vi "Main.vi"() -> ()   [LabVIEW 2010]
uses:
  <vilib>/Utility/inputDevices.llb/closeKeyboard.vi
  <vilib>/Utility/inputDevices.llb/keyboardAcquire.vi
panel:
  in  "Tab":enum32{"Load"}(tab)
  out "loading":u16(ring)
  in  "game show tab":T1(tab)=enum."Method"
  in  "Game Start":bool
  in  "Game Caption":bool
  in  "Game Restart":bool
  in  "String":string="1.按“SPACE”跳跃；\n2.按“SHIFT+SPACE”穿越障碍物！"
  in  "Game Sound":bool=TRUE
  in  "Game Pause":bool
  out "Load-I":i32=60
  in  "Game Close":bool
  in  "Game Slide":dbl(slide) scale=0.0..6.0
  in  "error in (no error)":errorcluster
  in  "MAP2":T2={"Game Road 1"=1, "Game Road 2"=1, "Game Road 3"=0, "Game Road 4"=1, "Game Road 5"=1, "Game Road 6"=1, "Game Road 7"=2, "Game Road 8"=1, "Game Road 9"=1, "Game Road 10"=1, "Game Road 11"=1, "Game Road 12"=1, "Game Road 13"=1, "Game Road 14"=1, "Game Road 15"=0, "Game Coin 1"=1, "Game Coin 2"=1, "Game Coin 3"=1, "Game Coin 4"=1, "Game Coin 5"=1, "Game Coin 6"=1, "Game Coin 7"=1, "Game Coin 8"=1, "Game Coin 9"=2, "Game Coin 10"=2, "Game Coin 11"=2, "Game Coin 12"=2, "Game Coin 13"=1, "Game Coin 14"=1, "Game Coin 15"=1, "Game Coin 16"=1, "Game Coin 17"=1, "Game Coin 18"=1, "Game Coin 19"=1, "Game Coin 20"=1, "Game Coin 21"=2, "Game Coin 22"=2, "Game Coin 23"=2, "Game Coin 24"=2, "Game Coin 25"=2, "Game Coin 26"=2, "Game Coin 27"=2, "Game Coin 28"=2, "Game Coin 29"=2, "Game Coin 30"=2, "Game Coin 31"=2, "Game Coin 32"=2, "Game Coin 33"=1, "Game Coin 34"=1, "Game Coin 35"=1, "Game Coin 36"=1, "Game Coin 37"=1, "Game Coin 38"=1, "Game Coin 39"=1, "Game Coin 40"=1, "Game Coin 41"=1, "Game Coin 42"=1, "Game Coin 43"=1, "Game Coin 44"=1, "Game Coin 45"=1, "Game Coin 46"=1, "Game Coin 47"=1, "Game Coin 48"=1, "Game Coin 49"=1, "Game Coin 50"=1, "Game Coin 51"=2, "Game Coin 52"=2, "Game Coin 53"=2, "Game Coin 54"=2, "Game Coin 55"=2, "Game Coin 56"=2, "Game Coin 57"=2, "Game Coin 58"=2, "Game Coin 59"=2, "Game Coin 60"=2}
  in  "Game Cat":u16(ring)=1
  out "Bool":bool
  in  "music":refnum<k7>(container)
  in  "background_music":refnum<k7>(container)
  in  "Score":u16[](array[ring])=[0, 0, 0, 0, 0, 0, 0, 0]
  in  "MAP1":T2={"Game Road 1"=1, "Game Road 2"=1, "Game Road 3"=1, "Game Road 4"=1, "Game Road 5"=1, "Game Road 6"=1, "Game Road 7"=0, "Game Road 8"=1, "Game Road 9"=1, "Game Road 10"=1, "Game Road 11"=1, "Game Road 12"=2, "Game Road 13"=1, "Game Road 14"=1, "Game Road 15"=0, "Game Coin 1"=0, "Game Coin 2"=0, "Game Coin 3"=0, "Game Coin 4"=0, "Game Coin 5"=1, "Game Coin 6"=1, "Game Coin 7"=1, "Game Coin 8"=1, "Game Coin 9"=1, "Game Coin 10"=1, "Game Coin 11"=1, "Game Coin 12"=1, "Game Coin 13"=1, "Game Coin 14"=1, "Game Coin 15"=1, "Game Coin 16"=1, "Game Coin 17"=1, "Game Coin 18"=1, "Game Coin 19"=1, "Game Coin 20"=1, "Game Coin 21"=1, "Game Coin 22"=1, "Game Coin 23"=1, "Game Coin 24"=2, "Game Coin 25"=2, "Game Coin 26"=2, "Game Coin 27"=2, "Game Coin 28"=2, "Game Coin 29"=2, "Game Coin 30"=1, "Game Coin 31"=1, "Game Coin 32"=1, "Game Coin 33"=1, "Game Coin 34"=1, "Game Coin 35"=1, "Game Coin 36"=1, "Game Coin 37"=1, "Game Coin 38"=1, "Game Coin 39"=1, "Game Coin 40"=2, "Game Coin 41"=2, "Game Coin 42"=2, "Game Coin 43"=2, "Game Coin 44"=1, "Game Coin 45"=1, "Game Coin 46"=1, "Game Coin 47"=1, "Game Coin 48"=1, "Game Coin 49"=1, "Game Coin 50"=2, "Game Coin 51"=2, "Game Coin 52"=2, "Game Coin 53"=2, "Game Coin 54"=2, "Game Coin 55"=2, "Game Coin 56"=2, "Game Coin 57"=2, "Game Coin 58"=2, "Game Coin 59"=2, "Game Coin 60"=2}
  in  "MAP3":T2={"Game Road 1"=1, "Game Road 2"=1, "Game Road 3"=1, "Game Road 4"=1, "Game Road 5"=1, "Game Road 6"=1, "Game Road 7"=0, "Game Road 8"=1, "Game Road 9"=1, "Game Road 10"=1, "Game Road 11"=2, "Game Road 12"=1, "Game Road 13"=1, "Game Road 14"=1, "Game Road 15"=0, "Game Coin 1"=1, "Game Coin 2"=1, "Game Coin 3"=1, "Game Coin 4"=1, "Game Coin 5"=1, "Game Coin 6"=1, "Game Coin 7"=1, "Game Coin 8"=1, "Game Coin 9"=1, "Game Coin 10"=1, "Game Coin 11"=1, "Game Coin 12"=1, "Game Coin 13"=1, "Game Coin 14"=1, "Game Coin 15"=1, "Game Coin 16"=1, "Game Coin 17"=1, "Game Coin 18"=1, "Game Coin 19"=1, "Game Coin 20"=1, "Game Coin 21"=1, "Game Coin 22"=1, "Game Coin 23"=1, "Game Coin 24"=2, "Game Coin 25"=2, "Game Coin 26"=2, "Game Coin 27"=2, "Game Coin 28"=2, "Game Coin 29"=2, "Game Coin 30"=2, "Game Coin 31"=1, "Game Coin 32"=1, "Game Coin 33"=1, "Game Coin 34"=1, "Game Coin 35"=1, "Game Coin 36"=1, "Game Coin 37"=1, "Game Coin 38"=1, "Game Coin 39"=1, "Game Coin 40"=1, "Game Coin 41"=2, "Game Coin 42"=2, "Game Coin 43"=2, "Game Coin 44"=2, "Game Coin 45"=1, "Game Coin 46"=1, "Game Coin 47"=1, "Game Coin 48"=1, "Game Coin 49"=1, "Game Coin 50"=1, "Game Coin 51"=1, "Game Coin 52"=1, "Game Coin 53"=1, "Game Coin 54"=1, "Game Coin 55"=2, "Game Coin 56"=2, "Game Coin 57"=2, "Game Coin 58"=2, "Game Coin 59"=2, "Game Coin 60"=2}
  in  "Game Cat head":u16(ring)=1
  out "Hscore":u16[](array[ring])=[0, 0, 0, 0, 5, 1, 5, 0]
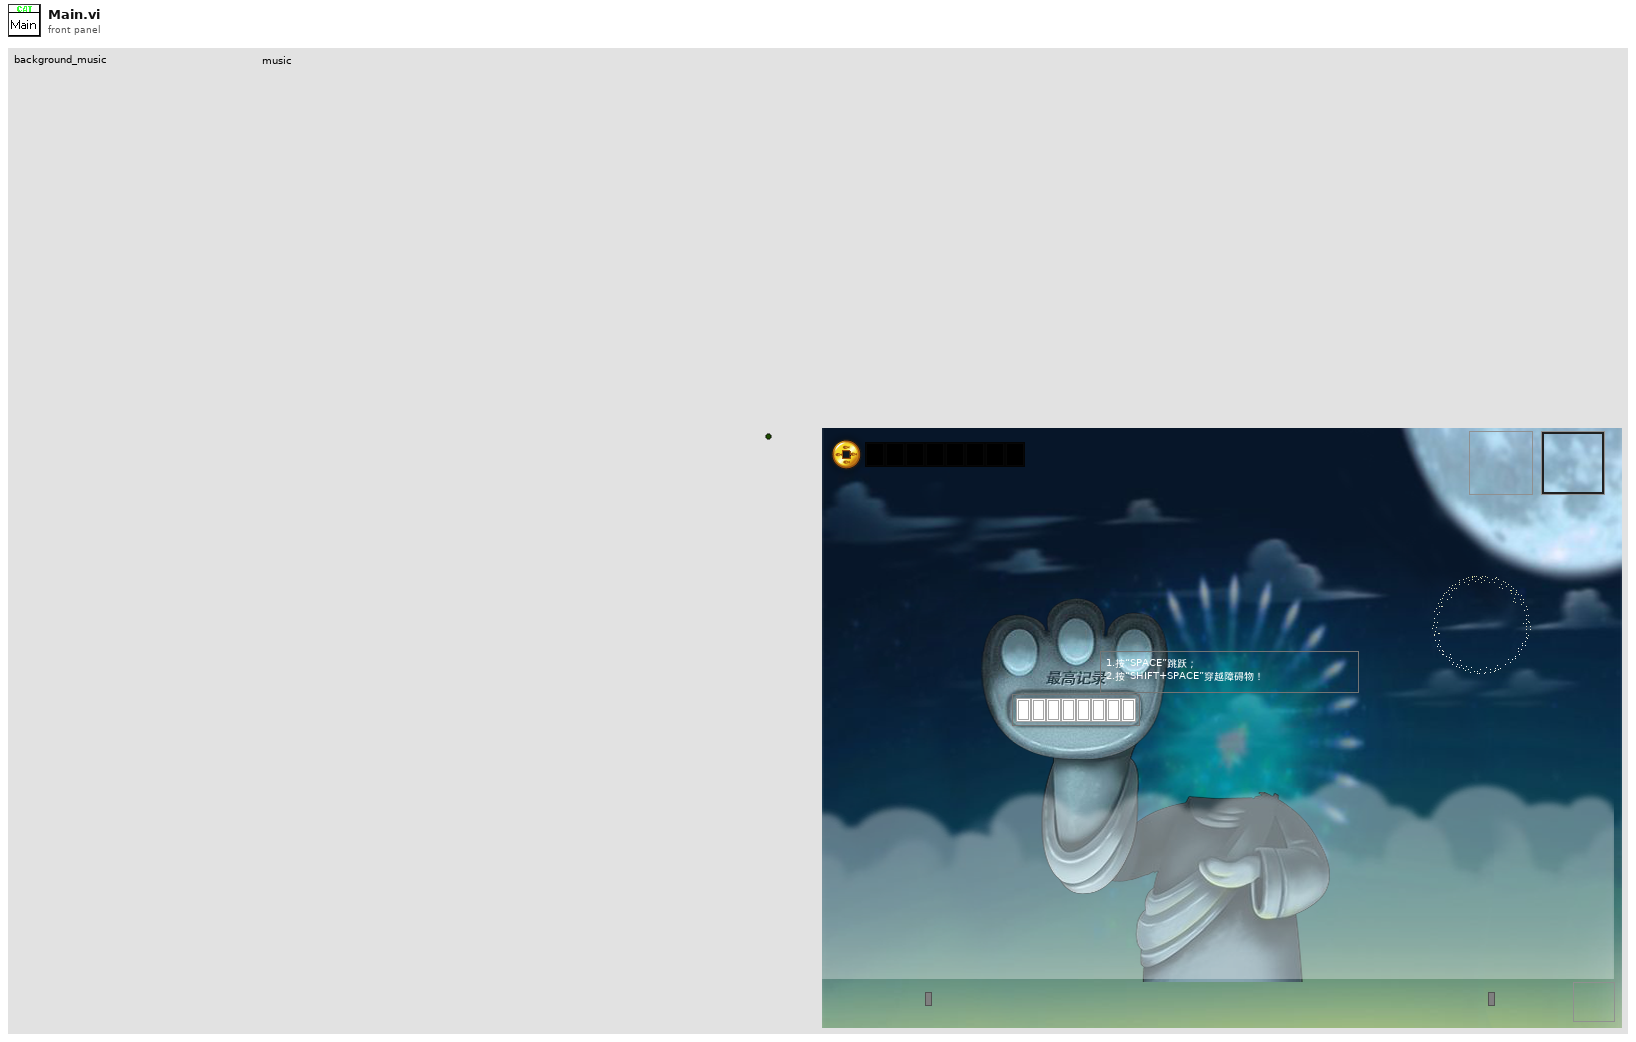
[diagram p1: front panel]
types:
  T1 = enum32{"Start", "Over", "Pause", "Game", "Method"}
  T2 = cluster{"Game Road 1":u16, "Game Road 2":u16, "Game Road 3":u16, "Game Road 4":u16, "Game Road 5":u16, "Game Road 6":u16, "Game Road 7":u16, "Game Road 8":u16, "Game Road 9":u16, "Game Road 10":u16, "Game Road 11":u16, "Game Road 12":u16, "Game Road 13":u16, "Game Road 14":u16, "Game Road 15":u16, "Game Coin 1":u16, "Game Coin 2":u16, "Game Coin 3":u16, "Game Coin 4":u16, "Game Coin 5":u16, "Game Coin 6":u16, "Game Coin 7":u16, "Game Coin 8":u16, "Game Coin 9":u16, "Game Coin 10":u16, "Game Coin 11":u16, "Game Coin 12":u16, "Game Coin 13":u16, "Game Coin 14":u16, "Game Coin 15":u16, "Game Coin 16":u16, "Game Coin 17":u16, "Game Coin 18":u16, "Game Coin 19":u16, "Game Coin 20":u16, "Game Coin 21":u16, "Game Coin 22":u16, "Game Coin 23":u16, "Game Coin 24":u16, "Game Coin 25":u16, "Game Coin 26":u16, "Game Coin 27":u16, "Game Coin 28":u16, "Game Coin 29":u16, "Game Coin 30":u16, "Game Coin 31":u16, "Game Coin 32":u16, "Game Coin 33":u16, "Game Coin 34":u16, "Game Coin 35":u16, "Game Coin 36":u16, "Game Coin 37":u16, "Game Coin 38":u16, "Game Coin 39":u16, "Game Coin 40":u16, "Game Coin 41":u16, "Game Coin 42":u16, "Game Coin 43":u16, "Game Coin 44":u16, "Game Coin 45":u16, "Game Coin 46":u16, "Game Coin 47":u16, "Game Coin 48":u16, "Game Coin 49":u16, "Game Coin 50":u16, "Game Coin 51":u16, "Game Coin 52":u16, "Game Coin 53":u16, "Game Coin 54":u16, "Game Coin 55":u16, "Game Coin 56":u16, "Game Coin 57":u16, "Game Coin 58":u16, "Game Coin 59":u16, "Game Coin 60":u16}
  T3 = enum16{"Init", "Game", "Over", "Finish", "Default"}
  T4 = enum8{"Enabled", "Disabled", "Disabled and Grayed Out"}
  T5 = enum16{"0", "1", "2", "3", "4", "5", "6", "7", "8", "9", "A", "B", "C", "D", "E", "F", "G", "H", "I", "J", "K", "L", "M", "N", "O", "P", "Q", "R", "S", "T", "U", "V", "W", "X", "Y", "Z", "F1", "F2", "F3", "F4", "F5", "F6", "F7", "F8", "F9", "F10", "F11", "F12", "F13", "F14", "F15", "ADD", "BACK", "BACKSLASH", "CAPITAL", "COMMA", "DECIMAL", "DELETE", "DIVIDE", "DOWN", "END", "EQUALS", "ESCAPE", "GRAVE (`)", "HOME", "INSERT", "LBRACKET", "LCONTROL", "LEFT", "L ALT", "LSHIFT", "LWIN", "MINUS", "MULTIPLY", "NEXT", "NUMLOCK", "NUMPAD_0", "NUMPAD_1", "NUMPAD_2", "NUMPAD_3", "NUMPAD_4", "NUMPAD_5", "NUMPAD_6", "NUMPAD_7", "NUMPAD_8", "NUMPAD_9", "PAUSE", "PERIOD", "PRIOR (PG UP)", "RBRACKET", "RCONTROL", "RETURN", "RIGHT", "R ALT", "RSHIFT", "RWIN", "SCROLL", "SEMICOLON", "SLASH", "SPACE", "SUBTRACT", "TAB", "UP", "ENTER (num pad)", "' (quote)"}[]
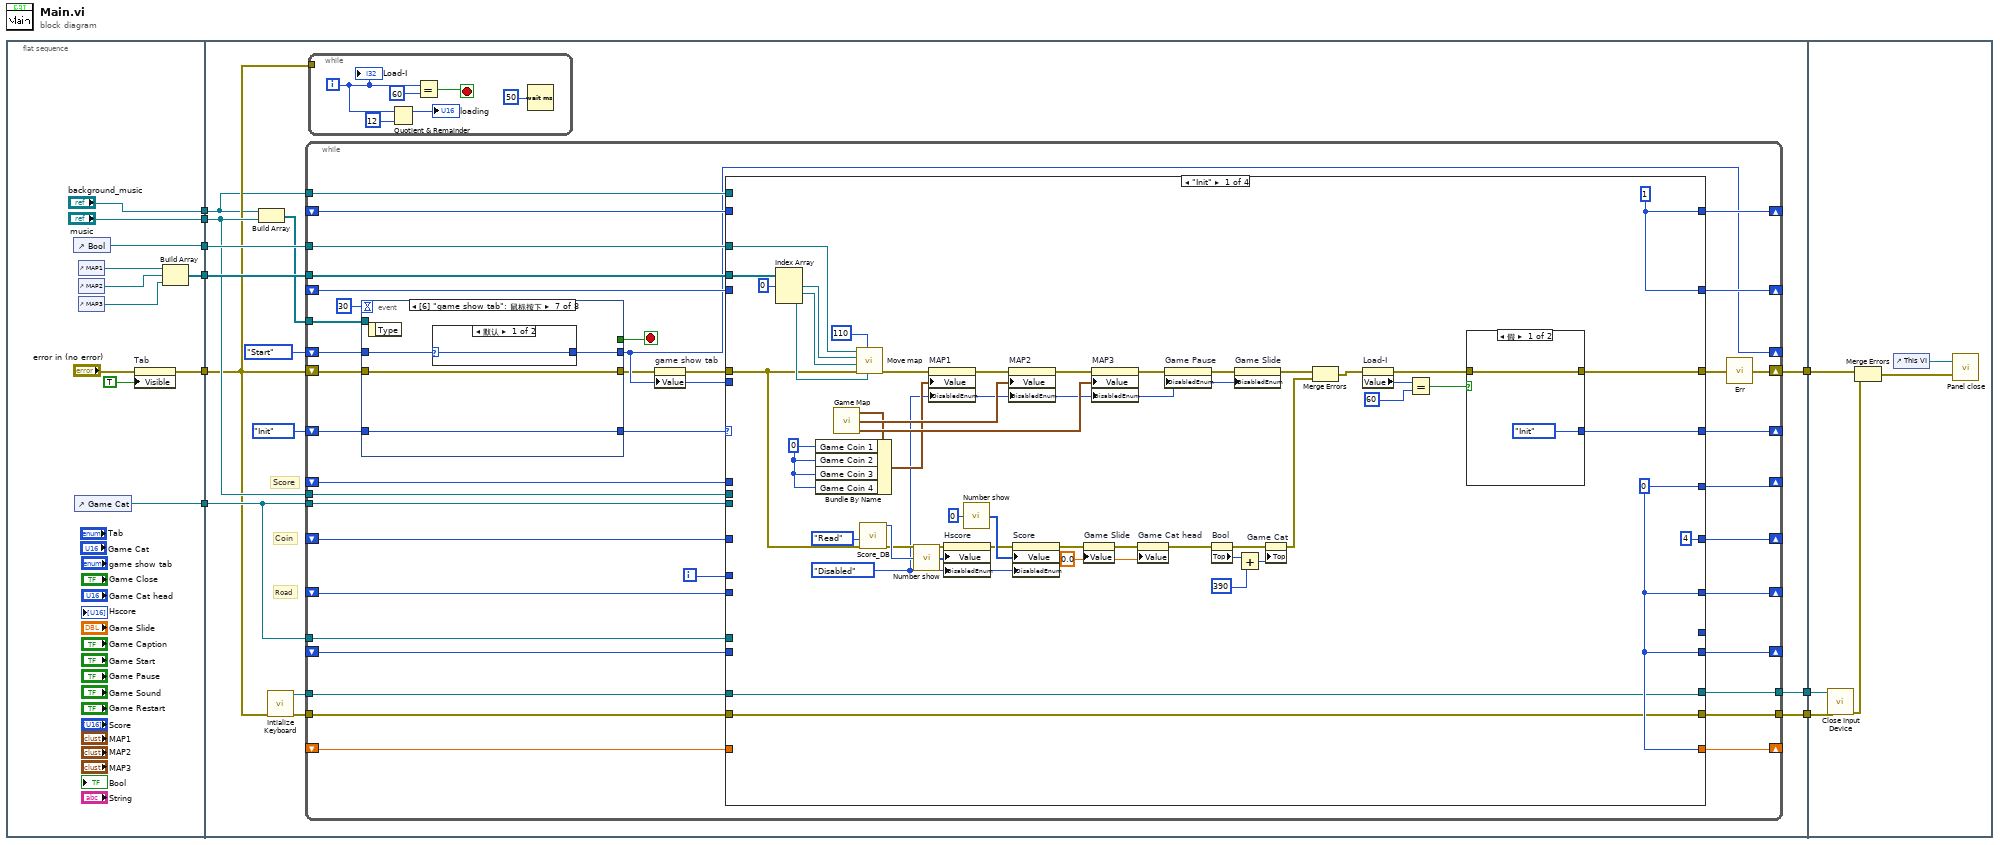
[diagram p0: block diagram]
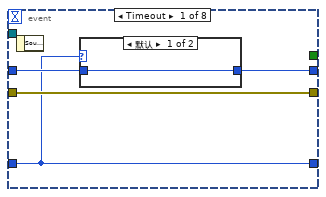
[diagram p2: hidden frame]
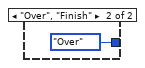
[diagram p3: hidden frame]
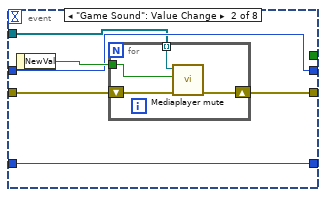
[diagram p4: hidden frame]
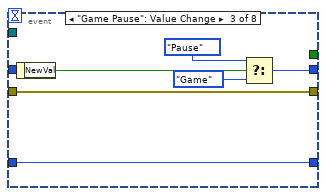
[diagram p5: hidden frame]
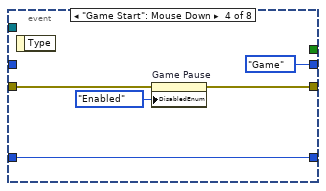
[diagram p6: hidden frame]
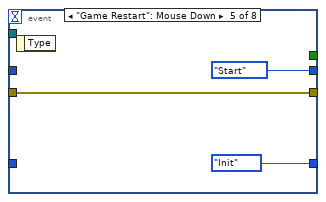
[diagram p7: hidden frame]
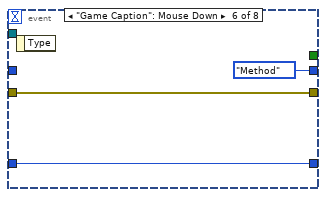
[diagram p8: hidden frame]
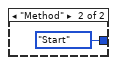
[diagram p9: hidden frame]
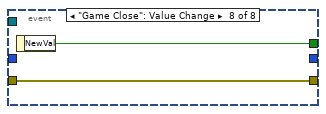
[diagram p10: hidden frame]
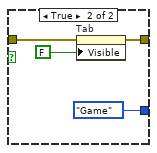
[diagram p11: hidden frame]
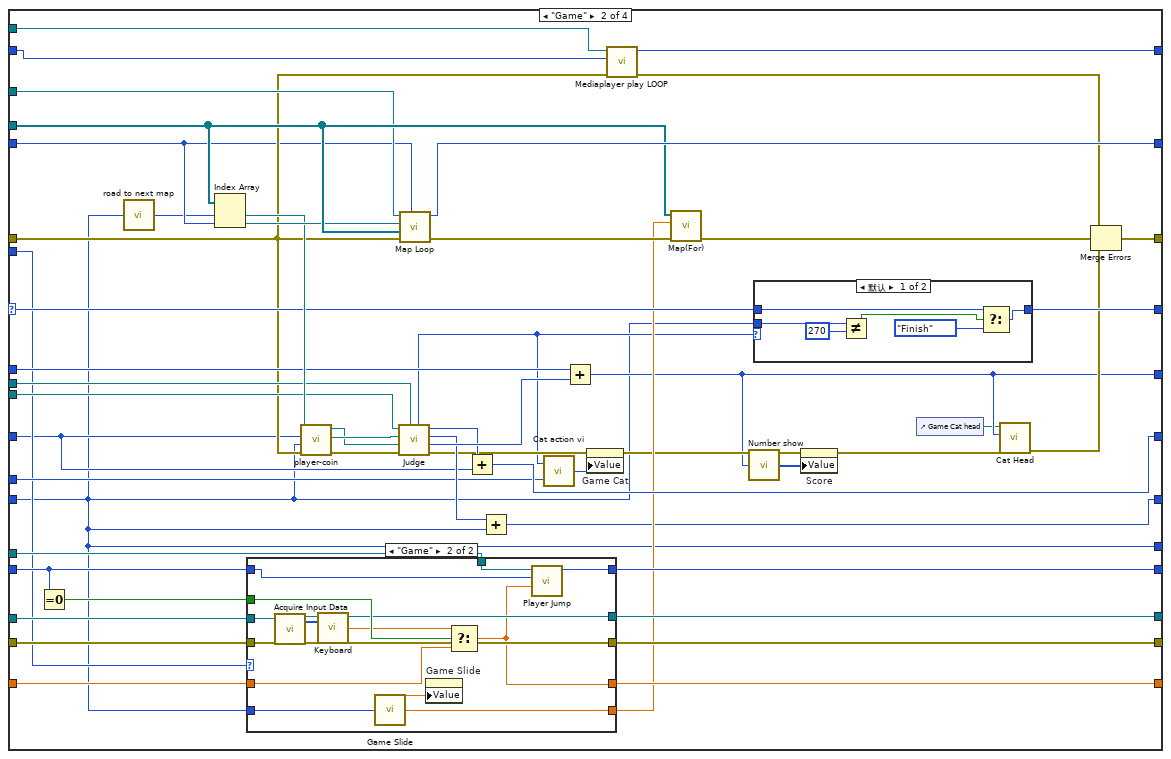
[diagram p12: hidden frame]
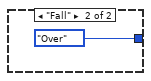
[diagram p13: hidden frame]
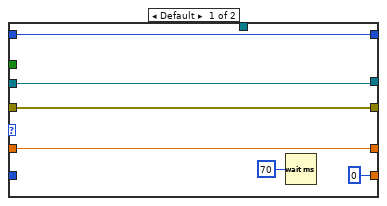
[diagram p14: hidden frame]
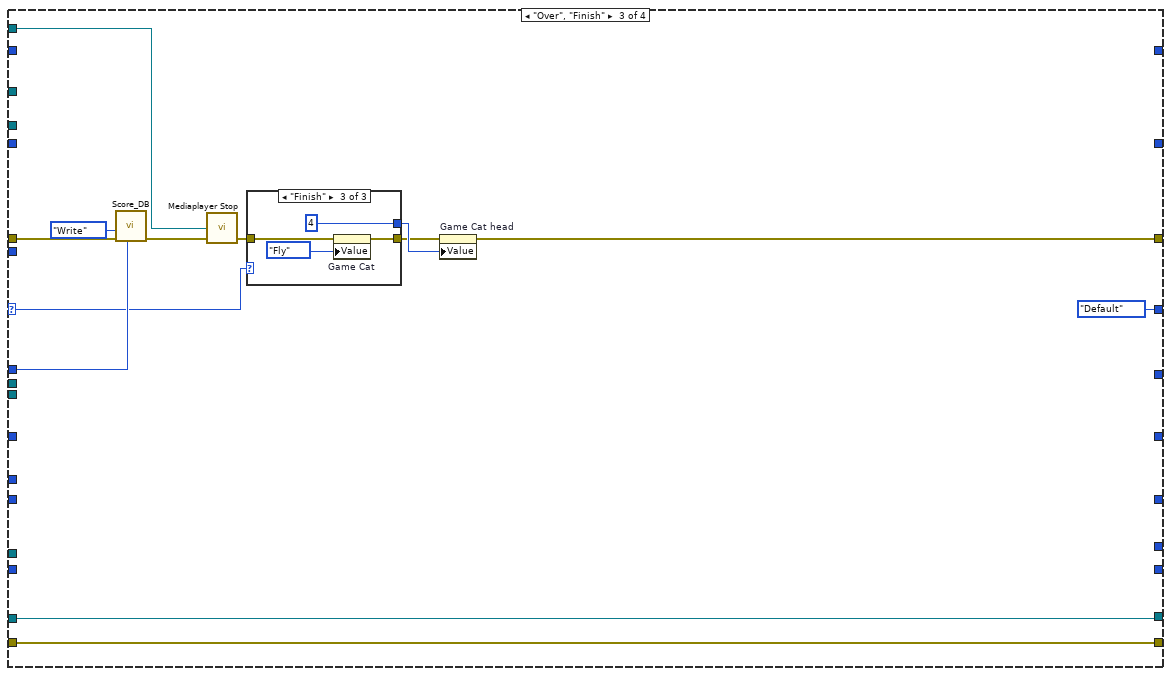
[diagram p15: hidden frame]
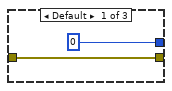
[diagram p16: hidden frame]
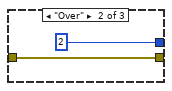
[diagram p17: hidden frame]
diagram:
  n1 = flat-sequence {
    tunnel: ["background_music"] -> w9
    tunnel: ["music"] -> w8
    tunnel: [w18] -> w7
    tunnel: [w17] -> w6
    tunnel: [w11] -> w5
    tunnel: [w10] -> w4
    tunnel: w9 -> [w24]
    tunnel: w8 -> [w32]
    tunnel: w7 -> [w34]
    tunnel: w6 -> [w33]
    tunnel: w5 -> [w30]
    tunnel: w4 -> [w31]
    tunnel: [w27] -> w3
    tunnel: [w26] -> w2
    tunnel: [w25] -> w1
    tunnel: w3 -> [w283]
    tunnel: w2 -> [w282]
    tunnel: w1 -> [w280]
    frame #0 {
      n2 = control-ref of="Bool"() -> (w18:refnum<vi>)
      n3 = control-ref of="Game Cat"() -> (w10:refnum<vi>)
      n4 = control-ref of="MAP1"() -> (w16:refnum<vi>)
      n5 = control-ref of="MAP2"() -> (w15:refnum<vi>)
      n6 = control-ref of="MAP3"() -> (w14:refnum<vi>)
      n7 = property on="Tab" class="TabCtl (严格)"(error in="error in (no error)", "Visible"=TRUE) -> (error out=w11:errorcluster)  [unwired: 1 in, 1 out]
      n8 = Build Array(w16, w15, w14) -> (w17:refnum<vi>[])
    }
    frame #1 {
      # "Score"
      # "Road"
      # "Coin"
      n9 = Build Array(w24, w32) -> (w22:refnum<k7>[])
      n10 = call <vilib>:"Intialize Keyboard.vi"("error in (no error)"=w30) -> ("error out"=w28:errorcluster, "device ID"=w29:refnum<k1>)  [unwired: 9 in]
      n11 = while {
        shift-right: [w77] -> _
        shift-left: _ -> [w78]
        shift-right: [w56] -> w25
        shift-left: w30 -> [w47]
        tunnel: w34 -> [w75]
        tunnel: w33 -> [w76]
        shift-right: [w51] -> _
        shift-left: T3."Init" ("State") -> [w45]
        shift-right: [w72] -> _
        shift-left: _ -> [w73]
        shift-right: [w71] -> _
        shift-left: _ -> [w70]
        shift-right: [w68] -> _
        shift-left: _ -> [w69]
        tunnel: w32 -> [w67]
        tunnel: w31 -> [w66]
        tunnel: w31 -> [w65]
        tunnel: w29 -> [w64]
        tunnel: w28 -> [w63]
        shift-right: [w62] -> _
        shift-left: _ -> [w61]
        shift-right: [w60] -> _
        shift-left: _ -> [w59]
        tunnel: [w58] -> w27
        tunnel: [w57] -> w26
        shift-right: [w54] -> _
        shift-left: _ -> [w53]
        tunnel: w24 -> [w52]
        shift-right: [w43] -> _
        shift-left: T1."Start" ("game show tab") -> [w49]
        tunnel: w22 -> [w48]
        i -> [w55]
        stop <- w46 stop-if-true
        n12 = event shown="[6] \"game show tab\": 鼠标按下" {
          selector: _ -> [_ _ _ _ _ _ _ _]
          dyn-events: _ -> [_ _ _ _ _ _ _ _]
          timeout: 30 -> [_ _ _ _ _ _ _ _]
          tunnel: w49 -> [w82 w89 _ _ _ _ w114 _]
          tunnel: [w81 w89 w98 T1."Game" ("game show tab") T1."Start" ("game show tab") T1."Method" ("game show tab") w115 _] -> w43
          tunnel: [_ _ _ _ _ _ _ w119] -> w46
          tunnel: w48 -> [_ w88 _ _ _ _ _ _]
          tunnel: w47 -> [w80 w87 w96 w103 w107 w109 w112 w118]
          tunnel: [w80 w86 w96 w102 w107 w109 w112 w118] -> w42
          tunnel: w45 -> [w79 w85 w95 w101 _ w110 w113 _]
          tunnel: [w79 w85 w95 w101 enum16{"Init", "Game", "Over", "Finish"}."Init" ("State") w110 w113 _] -> w44
          event Timeout {
            n13 = event-data() -> ()  [unwired: 1 in, 1 out]
            n14 = case shown="默认" w79 {
              tunnel: w82 -> [w83 _]
              tunnel: [w83 T1."Over" ("game show tab")] -> w81
              frame Default {
              }
              frame "Over", "Finish" {
              }
            }
          }
          event "Game Sound": Value Change {
            n15 = event-data() -> ("NewVal"=w90:bool)  [unwired: 1 in]
            n16 = for {
              tunnel: w90 -> [w94]
              shift-right: [w92] -> w86
              shift-left: w87 -> [w93]
              tunnel: w88 -> [w91] mode=indexing
              n17 = call "Mediaplayer mute.vi"("error in (no error)"=w93, "mute"=w94, "Refnum"=w91) -> ("error out"=w92:errorcluster)  [unwired: 8 in]
            }
          }
          event "Game Pause": Value Change {
            n18 = event-data() -> ("NewVal"=w100:bool)  [unwired: 1 in]
            n19 = Select(t=T1."Pause" ("game show tab"), s=w100, f=T1."Game") -> (s? t:f=w98:T1)
          }
          event "Game Start": Mouse Down {
            n20 = event-data() -> ()  [unwired: 1 in, 1 out]
            n21 = property on="Game Pause" class="Bool (严格)"(error in=w103, "DisabledEnum"=T4."Enabled" ("Disabled")) -> (error out=w102:errorcluster)  [unwired: 1 in, 1 out]
          }
          event "Game Restart": Mouse Down {
            n22 = event-data() -> ()  [unwired: 1 in, 1 out]
          }
          event "Game Caption": Mouse Down {
            n23 = event-data() -> ()  [unwired: 1 in, 1 out]
          }
          event "game show tab": Mouse Down {
            n24 = event-data() -> ()  [unwired: 1 in, 1 out]
            n25 = case shown="默认" w114 {
              selector: w114 -> [w116 _]
              tunnel: [w116 T1."Start" ("game show tab")] -> w115
              frame Default {
              }
              frame "Method" {
              }
            }
          }
          event "Game Close": Value Change {
            n26 = event-data() -> ("NewVal"=w119:bool)  [unwired: 1 in]
          }
        }
        n27 = property on="game show tab" class="TabCtl (严格)"(error in=w42, "Value"=w43) -> (error out=w41:errorcluster)  [unwired: 1 in, 1 out]
        n28 = case shown="\"Init\"" w44 {
          selector: w44 -> [_ w199 w258 w275]
          tunnel: w78 -> [_ w176 _ _]
          tunnel: [w134 w225 _ _] -> w77
          tunnel: w76 -> [w158 w224 _ _]
          tunnel: w75 -> [w154 w223 _ _]
          tunnel: [w145 w196 w261 w276] -> w74
          tunnel: w41 -> [w128 w179 w266 w276]
          tunnel: [w144 w198 T3."Default" ("State") w275] -> w51
          tunnel: w73 -> [_ w177 _ _]
          tunnel: [4 w213 _ _] -> w72
          tunnel: [w129 w194 _ _] -> w71
          tunnel: w70 -> [_ w175 _ _]
          tunnel: w69 -> [_ w217 w264 _]
          tunnel: [w129 w180 _ _] -> w68
          tunnel: w67 -> [_ w200 _ _]
          tunnel: w66 -> [_ w211 _ _]
          tunnel: w65 -> [_ w204 _ _]
          tunnel: w64 -> [w125 w210 w260 w277]
          tunnel: w63 -> [w124 w209 w259 w278]
          tunnel: [w129 w202 _ _] -> w62
          tunnel: w61 -> [_ w203 _ _]
          tunnel: [w129 w201 _ _] -> w60
          tunnel: w59 -> [_ w207 _ _]
          tunnel: [w125 w206 w260 w277] -> w58
          tunnel: [w124 w205 w259 w278] -> w57
          tunnel: [_ w175 _ _] -> _
          tunnel: w55 -> [_ w189 _ _]
          tunnel: [w134 w188 _ _] -> w54
          tunnel: w53 -> [_ w185 _ _]
          tunnel: w52 -> [_ w187 w262 _]
          tunnel: w43 -> [_ w184 _ _]
          frame "Init" {
            w133 = 0.0 ("Game Slide")
            w120 = T4."Disabled" ("Disabled")
            w139 = u16 0 ("Game Coin 1")
            w129 = u16 0
            w134 = 1
            n29 = Index Array(array=w158, index #1=0 ("index")) -> (element #1=w157:refnum<vi>, element #2=w156:refnum<vi>, element #3=w155:refnum<vi>)  [unwired: 2 in]
            n30 = call "Game Map.vi"() -> ("MAP1"=w148:T2, "MAP2"=w164:T2, "MAP3"=w163:T2)  [unwired: 5 in]
            n31 = Bundle By Name(cluster=w148, "Game Coin 1"=w139, "Game Coin 2"=w139, "Game Coin 3"=w139, "Game Coin 4"=w139) -> (w147:T2)
            n32 = call "Move map.vi"("MAP3"=w155, "revise"=u32 110, "error in"=w128, "MAP2"=w156, "MAP1"=w157, "Boolean in"=w154) -> ("error out"=w153:errorcluster)  [unwired: 5 in]
            n33 = call "Score_DB.vi"("error in (no error)"=w128, "Enum"=enum16{"Read", "Write"}."Read") -> ("error out"=w165:errorcluster, "max score"=w166:i32)  [unwired: 7 in]
            n34 = call "Number show.vi"("Numeric"=w166) -> ("Number Array"=w167:u16[])  [unwired: 14 in]
            n35 = property on="MAP1" class="Clust (严格)"(error in=w153, "Value"=w147, "DisabledEnum"=w120) -> (error out=w152:errorcluster)  [unwired: 1 in, 1 out]
            n36 = property on="Hscore" class="Arr (严格)"(error in=w165, "Value"=w167, "DisabledEnum"=w120) -> (error out=w160:errorcluster)  [unwired: 1 in, 1 out]
            n37 = call "Number show.vi"("Numeric"=u32 0) -> ("Number Array"=w161:u16[])  [unwired: 14 in]
            n38 = property on="MAP2" class="Clust (严格)"(error in=w152, "Value"=w164, "DisabledEnum"=w120) -> (error out=w151:errorcluster)  [unwired: 1 in, 1 out]
            n39 = property on="Score" class="Arr (严格)"(error in=w160, "Value"=w161, "DisabledEnum"=w120) -> (error out=w131:errorcluster)  [unwired: 1 in, 1 out]
            n40 = property on="Game Slide" class="Slide (严格)"(error in=w131, "Value"=w133) -> (error out=w132:errorcluster)  [unwired: 1 in, 1 out]
            n41 = property on="MAP3" class="Clust (严格)"(error in=w151, "Value"=w163, "DisabledEnum"=w120) -> (error out=w146:errorcluster)  [unwired: 1 in, 1 out]
            n42 = property on="Game Cat head" class="Ring (严格)"(error in=w132, "Value"=w133) -> (error out=w130:errorcluster)  [unwired: 1 in, 1 out]
            n43 = property on="Game Pause" class="Bool (严格)"(error in=w146, "DisabledEnum"=w120) -> (error out=w122:errorcluster)  [unwired: 1 in, 1 out]
            n44 = property on="Bool" class="Bool (严格)"(error in=w130) -> (error out=w138:errorcluster, "Top"=w137:i32)  [unwired: 1 in, 1 out]
            n45 = property on="Game Slide" class="Slide (严格)"(error in=w122, "DisabledEnum"=w120) -> (error out=w121:errorcluster)  [unwired: 1 in, 1 out]
            n46 = Add(x=w137, y=390) -> (x+y=w136:i32)
            n47 = property on="Game Cat" class="Ring (严格)"(error in=w138, "Top"=w136) -> (error out=w127:errorcluster)  [unwired: 1 in, 1 out]
            n48 = Merge Errors(w121, w127) -> (w126:errorcluster)
            n49 = property on="Load-I" class="DigNum (严格)"(error in=w126) -> (error out=w143:errorcluster, "Value"=w141:i32)  [unwired: 1 in, 1 out]
            n50 = Equal?(x=w141, y=60) -> (x = y?=w142:bool)
            n51 = case shown="假" w142 {
              tunnel: w143 -> [w169 w172]
              tunnel: [w169 w171] -> w145
              tunnel: [T3."Init" ("State") T3."Game" ("State")] -> w144
              frame False {
              }
              frame True {
                n52 = property on="Tab" class="TabCtl (严格)"(error in=w172, "Visible"=FALSE) -> (error out=w171:errorcluster)  [unwired: 1 in, 1 out]
              }
            }
          }
          frame "Game" {
            n53 = Equal To 0?(x=w203) -> (x = 0?=w208:bool)
            n54 = call "road to next map.vi"("Numeric in"=w175) -> ("Numeric out"=w174:i32)  [unwired: 14 in]
            n55 = Index Array(array=w224, index #1=w174, index #2=w176) -> (element #1=w220:refnum<vi>, element #2=w221:refnum<vi>)
            n56 = case shown="\"Game\"" w184 {
              tunnel: w210 -> [w238 w253]
              tunnel: w209 -> [w237 w252]
              tunnel: [w236 w242] -> w201
              tunnel: w208 -> [_ w250]
              tunnel: w207 -> [w236 w248]
              tunnel: [w238 w247] -> w206
              tunnel: [w237 w246] -> w205
              tunnel: w204 -> [_ w245]
              tunnel: w203 -> [w235 w244]
              tunnel: [w235 w243] -> w202
              tunnel: [0 w241] -> w195
              tunnel: w175 -> [_ w240]
              frame Default {
                n57 = Wait (ms)(milliseconds to wait=u32 70) -> ()  [unwired: 1 out]
              }
              frame "Game" {
                n58 = call-poly <vilib>:"Acquire Input Data.vi"("device ID"=w253, "error in (no error)"=w252) -> ("device ID"=w247:refnum<k1>, "keys pressed"=w251:T5, "error out"=w246:errorcluster)  [unwired: 15 in]
                n59 = call "Keyboard.vi"("Array"=w251) -> ("step"=w249:dbl)  [unwired: 14 in]
                n60 = call "Game Slide.vi"("Numeric in"=w240) -> ("Game Slide"=w239:dbl, "Step"=w241:dbl)  [unwired: 13 in]
                n61 = property on="Game Slide" class="Slide (严格)"("Value"=w239) -> ()  [unwired: 2 in, 2 out]
                n62 = Select(t=w249, s=w250, f=w248) -> (s? t:f=w242:dbl)
                n63 = call "Player Jump.vi"("step"=w242, "Numeric in"=w244, "Ring in"=w245) -> ("Numeric out"=w243:u16)  [unwired: 7 in, 1 out]
              }
            }
            n64 = call "player-coin.vi"("error in (no error)"=w179, "Game Road Numeric"=w175, "Game Coin Numeric"=w177, "Cluster"=w220) -> ("error out"=w183:errorcluster, "Game Coin Ref"=w219:refnum<vi>, "Game Road Ref"=w218:refnum<vi>)  [unwired: 5 in]
            n65 = call "Judge.vi"("mediaplayer"=w200, "error in (no error)"=w183, "Road Refnum"=w218, "Coin Refnum"=w219, "Player Refnum"=w211) -> ("error out"=w192:errorcluster, "Score"=w216:u16, "roadnext"=w214:i32, "coinnext"=w215:i32, "Action"=w190:enum16{"Cat", "Jump", "Fall", "Fly", "Rote"})  [unwired: 1 in]
            n66 = call "Map Loop.vi"("I in"=w176, "error in (no error)"=w179, "Array"=w224, "MAP"=w221, "Boolean in"=w223) -> ("error out"=w222:errorcluster, "I next out"=w225:i64)  [unwired: 5 in]
            n67 = Add(x=w215, y=w177) -> (x+y=w213:i32)
            n68 = Add(x=w214, y=w175) -> (x+y=w194:i32)
            n69 = call "Cat action vi.vi"("i"=w189, "Action"=w190) -> ("Game Cat"=w193:u16)
            n70 = Add(x=w217, y=w216) -> (x+y=w180:u16)
            n71 = property on="Game Cat" class="Ring (严格)"(error in=w192, "Value"=w193) -> (error out=w191:errorcluster)  [unwired: 1 in, 1 out]
            n72 = call "Mediaplayer play LOOP.vi"("error in (no error)"=w179, "playState in"=w185, "Automation Refnum in"=w187) -> ("error out"=w186:errorcluster, "playState out"=w188:i32)  [unwired: 7 in]
            n73 = call "Map(For).vi"("error in (no error)"=w222, "Step"=w195, "Map"=w224) -> ("error out"=w197:errorcluster)  [unwired: 8 in]
            n74 = call "Number show.vi"("Numeric"=w180) -> ("Number Array"=w212:u16[])  [unwired: 14 in]
            n75 = case shown="默认" w190 {
              tunnel: w199 -> [w230 _]
              tunnel: [w231 T3."Over" ("State")] -> w198
              tunnel: w175 -> [w229 _]
              frame Default {
                n76 = Not Equal?(x=w229, y=270) -> (x != y?=w228:bool)
                n77 = Select(t=w230, s=w228, f=T3."Finish" ("State")) -> (s? t:f=w231:T3)
              }
              frame "Fall" {
              }
            }
            n78 = property on="Score" class="Arr (严格)"(error in=w191, "Value"=w212) -> (error out=w182:errorcluster)  [unwired: 1 in, 1 out]
            n79 = control-ref of="Game Cat head"() -> (w178:refnum<vi>)
            n80 = call "Cat Head.vi"("error in (no error)"=w182, "Numeric"=w180, "Ring in"=w178) -> ("error out"=w181:errorcluster)  [unwired: 8 in]
            n81 = Merge Errors(w186, w197, w181) -> (w196:errorcluster)
          }
          frame "Over", "Finish" {
            n82 = call "Score_DB.vi"("Score"=w264, "error in (no error)"=w266, "Enum"=enum16{"Read", "Write"}."Write") -> ("error out"=w263:errorcluster)  [unwired: 6 in, 1 out]
            n83 = call "Mediaplayer Stop.vi"("MediaPlayer"=w262, "error in"=w263) -> ("error out"=w256:errorcluster)  [unwired: 5 in]
            n84 = case shown="\"Finish\"" w258 {
              tunnel: [u16 0 ("Game Cat head") u16 2 ("Game Cat head") u16 4 ("Game Cat head")] -> w257
              tunnel: w256 -> [w267 w269 w272]
              tunnel: [w267 w269 w271] -> w255
              frame Default {
              }
              frame "Over" {
              }
              frame "Finish" {
                n85 = property on="Game Cat" class="Ring (严格)"(error in=w272, "Value"=enum16{"Cat", "Jump", "Fall", "Fly", "Rote"}."Fly" ("Action")) -> (error out=w271:errorcluster)  [unwired: 1 in, 1 out]
              }
            }
            n86 = property on="Game Cat head" class="Ring (严格)"(error in=w255, "Value"=w257) -> (error out=w261:errorcluster)  [unwired: 1 in, 1 out]
          }
          frame Default {
          }
        }
        n87 = call "Err.vi"("error in"=w74) -> ("error out"=w56:errorcluster)
      }
      n88 = while {
        tunnel: w30 -> [_]
        i -> [w35]
        stop <- w36 stop-if-true
        n89 = Quotient & Remainder(x=w35, y=12) -> (x-y*floor(x/y)=→"loading":i32)  [unwired: 1 out]
        n90 = Equal?(x=w35, y=60) -> (x = y?=w36:bool)
        n91 = Wait (ms)(milliseconds to wait=u32 50) -> ()  [unwired: 1 out]
        "Load-I" <- w35
      }
    }
    frame #2 {
      n92 = call-poly <vilib>:"Close Input Device.vi"("error in (no error)"=w282, "device ID"=w283) -> ("error out"=w279:errorcluster)  [unwired: 8 in]
      n93 = Merge Errors(w280, w279) -> (w281:errorcluster)
      n94 = control-ref of="This VI"() -> (w284:refnum<vi>)
      n95 = call "Panel close.vi"("error in"=w281, "This VI"=w284) -> ()  [unwired: 1 in, 1 out]
    }
  }
